vi "Teil Array speichern.vi"(0 "Komplette Datei":string[][](array[string]), 5 "AK NAME Teil":string[][](array[string]), 9 "EKFG Teil":string[][](array[string]), 11 "error in (no error)":errorcluster caption="Fehler (Eingang, kein Fehler)", 13 "Aktion":T1) -> (4 "Komplette Datei":string[][](array[string]), 6 "Rezpt nicht gefunden":bool, 8 "END nicht gefunden":bool, 15 "error out":errorcluster caption="Fehler (Ausgang)")   [LabVIEW 2020, in "AK-Schnittstelle.lvlib"]
uses:
  AK-Schnittstelle.lvlib
  Aktion Array speichern.ctl
  Stoerungen/Stoerungen Messgeraet/Aktionen Kommunikation Stoerung.ctl
  Seiten/FT-IR/FGV FT-IR Aktionen.ctl
  Stoerungen/Stoerungen.lvlib
  Seiten/FT-IR/FT-IR.lvlib
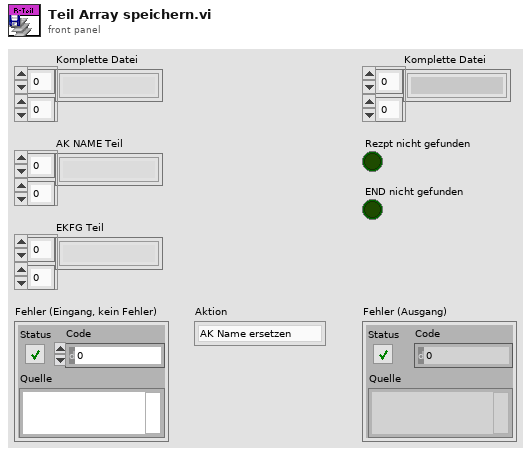
[diagram p1: front panel]
types:
  T1 = typedef "AK-Schnittstelle.lvlib/Aktion Array speichern.ctl" = enum16{"AK Name ersetzen", "EKFG ersetzen", "Rezept fehler", "neues Rezept erstellen"}
  T2 = typedef "FT-IR.lvlib/FGV FT-IR Aktionen.ctl" = enum16{"lesen", "NOG setzen", "NOS setzen", "Initialisieren", "speichern", "ALLES setzen", "FT-IR Spektrum loggen", "Komm Stoppen", "Spektrum LogKonfig"}
  T3 = typedef "Stoerungen.lvlib/Aktionen Kommunikation Stoerung.ctl" = enum16{"lesen", "init", "FT-IR Komm", "FT-IR Betriebsart", "FT-IR Hintergrund", "cRIO Komm", "PNS Komm", "Dichtheitstest", "Life Bit", "FTIR Komm AK", "PMA Komm", "FID Komm", "PMA Cal", "FID Ch4 Cal", "FID THC Cal", "Cal Timeout", "VFS 1 Komm", "VFS 2 Komm", "VFS 3 Komm", "VFS 4 Komm", "TRE 08 Komm", "CG-Test vorzeitig", "CG-Test Span 1", "CG-Test Span 2", "CG-Test Span 3", "CG-Test Messgas", "CG-Test löschen", "Test", "Amium AK", "AK Recept konfig", "AK Name konfig", "AK EKFG konfig"}
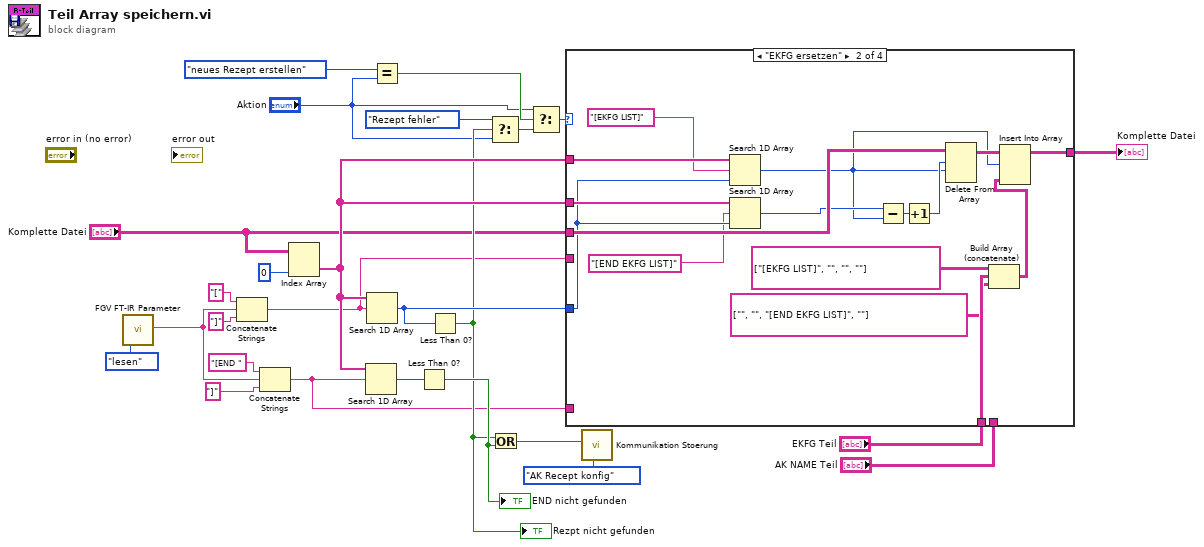
[diagram p0: block diagram]
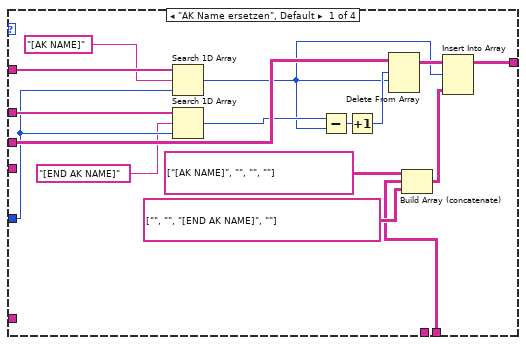
[diagram p2: hidden frame]
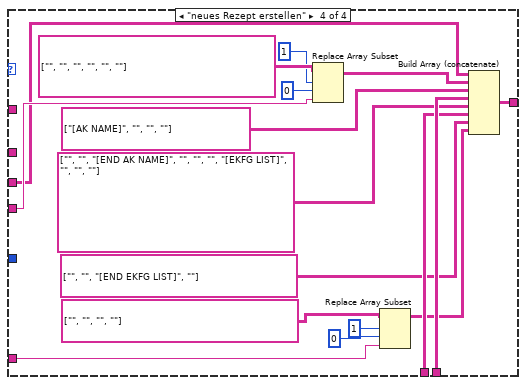
[diagram p4: hidden frame]
diagram:
  n1 = call "FGV FT-IR Parameter.vi"("Aktion"=FGV_FT-IR_Aktionen."lesen") -> ("Current Recipe"=w4:string)  [unwired: 11 in, 7 out]
  n2 = Concatenate Strings("[" ("String"), w4, "]" ("String")) -> (w3:string)
  n3 = Concatenate Strings("[END " ("String"), w4, "]" ("String")) -> (w1:string)
  n4 = Index Array(array="Komplette Datei", index (col)=0 ("Deaktivierter Index (Spalte)")) -> (element=w14:string[])  [unwired: 1 in]
  n5 = Search 1D Array(1D array=w14, element=w1) -> (index of element=w21:i32)  [unwired: 1 in]
  n6 = Search 1D Array(1D array=w14, element=w3) -> (index of element=w15:i32)  [unwired: 1 in]
  n7 = Equal?(x=Aktion_Array_speichern."neues Rezept erstellen" ("Aktion"), y="Aktion") -> (x = y?=w6:bool)
  n8 = Less Than 0?(x=w21) -> (x < 0?=w18:bool)
  "END nicht gefunden" <- w18
  n9 = Less Than 0?(x=w15) -> (x < 0?=w13:bool)
  "Rezpt nicht gefunden" <- w13
  n10 = Select(t=Aktion_Array_speichern."Rezept fehler" ("Aktion"), s=w13, f="Aktion") -> (s? t:f=w8:T1)
  n11 = Or(x=w13, y=w18) -> (x .or. y?=w19:bool)
  n12 = Select(t="Aktion", s=w6, f=w8) -> (s? t:f=w7:T1)
  n13 = case shown="\"EKFG ersetzen\"" w7 {
    tunnel: "Komplette Datei" -> [w39 w55 w59 w60]
    tunnel: [w38 w54 w59 w66] -> w16
    tunnel: w14 -> [w37 w53 _ _]
    tunnel: w15 -> [w33 w49 _ _]
    tunnel: w14 -> [w36 w52 _ _]
    tunnel: "AK NAME Teil" -> [w27 _ _ w73]
    tunnel: "EKFG Teil" -> [_ w45 _ w71]
    tunnel: w3 -> [_ _ _ w70]
    tunnel: w1 -> [_ _ _ w62]
    frame "AK Name ersetzen", Default {
      n14 = Search 1D Array(1D array=w36, element="[AK NAME]" ("String"), start index (0)=w33) -> (index of element=w34:i32)
      n15 = Search 1D Array(1D array=w37, element="[END AK NAME]" ("String"), start index (0)=w33) -> (index of element=w35:i32)
      n16 = Subtract(x=w35, y=w34) -> (x-y=w42:i32)
      n17 = Increment(x=w42) -> (x+1=w41:i32)
      n18 = Delete From Array(array=w39, length=w41, index (row)=w34) -> (array with subset deleted=w40:string[][])  [unwired: 1 in, 1 out]
      n19 = Build Array (concatenate)(string[][] [["[AK NAME]", ""], ["", ""]], w27, string[][] [["", ""], ["[END AK NAME]", ""]]) -> (w28:string[][])
      n20 = Insert Into Array(array=w40, index (row)=w34, new element=w28) -> (w38:string[][])  [unwired: 1 in]
    }
    frame "EKFG ersetzen" {
      n21 = Search 1D Array(1D array=w52, element="[EKFG LIST]" ("String"), start index (0)=w49) -> (index of element=w50:i32)
      n22 = Search 1D Array(1D array=w53, element="[END EKFG LIST]" ("String"), start index (0)=w49) -> (index of element=w51:i32)
      n23 = Subtract(x=w51, y=w50) -> (x-y=w58:i32)
      n24 = Increment(x=w58) -> (x+1=w57:i32)
      n25 = Delete From Array(array=w55, length=w57, index (row)=w50) -> (array with subset deleted=w56:string[][])  [unwired: 1 in, 1 out]
      n26 = Build Array (concatenate)(string[][] [["[EKFG LIST]", ""], ["", ""]], w45, string[][] [["", ""], ["[END EKFG LIST]", ""]]) -> (w43:string[][])
      n27 = Insert Into Array(array=w56, index (row)=w50, new element=w43) -> (w54:string[][])  [unwired: 1 in]
    }
    frame "Rezept fehler" {
    }
    frame "neues Rezept erstellen" {
      n28 = Replace Array Subset(array=string[][] [["", ""], ["", ""], ["", ""]], new element=w70, index (row)=1 ("Index (Zeile)"), index (col)=0 ("Index (Zeile)")) -> (w75:string[][])
      n29 = Replace Array Subset(array=string[][] [["", ""], ["", ""]], new element=w62, index (row)=1 ("Index (Zeile)"), index (col)=0 ("Index (Zeile)")) -> (w61:string[][])
      n30 = Build Array (concatenate)(w60, w75, string[][] [["[AK NAME]", ""], ["", ""]], w73, string[][] [["", ""], ["[END AK NAME]", ""], ["", ""], ["[EKFG LIST]", ""], ["", ""]], w71, string[][] [["", ""], ["[END EKFG LIST]", ""]], w61) -> (w66:string[][])
    }
  }
  "Komplette Datei" <- w16
  n31 = call "Kommunikation Stoerung.vi"("Aktionen"=Aktionen_Kommunikation_Stoerung."AK Recept konfig", "ERROR"=w19) -> ()  [unwired: 9 in, 1 out]
